vi "Configure Averaging.vi"(5 "Averaging State (F: Off)":bool, 7 "Channel (1)":i32=1, 8 "error in (no error)":errorcluster, 10 "Factor (16)":i32=16, 11 "VISA resource name":refnum<visa-resource-name>) -> (0 "error out":errorcluster, 3 "VISA resource name out":refnum<visa-resource-name>)   [LabVIEW 2011, in "Agilent ENA Series.lvlib"]
doc: "This VI configure the averaging for active channel."
uses:
  Agilent ENA Series.lvlib
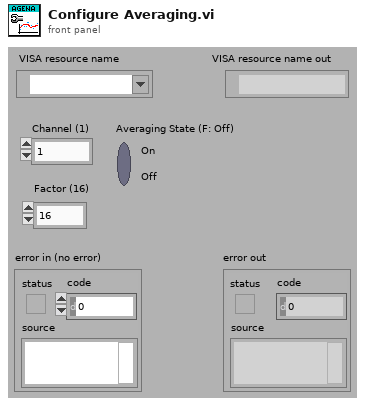
[diagram p1: front panel]
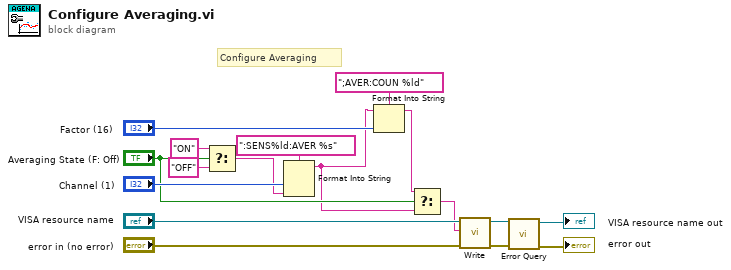
[diagram p0: block diagram]
diagram:
  # "Configure Averaging"
  n1 = Select(t="ON", s="Averaging State (F: Off)", f="OFF") -> (s? t:f=w11:string)
  n2 = Format Into String(format string=":SENS%ld:AVER %s", "Channel (1)", w11) -> (resulting string=w5:string)  [unwired: 2 in, 1 out]
  n3 = Format Into String(format string=";AVER:COUN %ld", initial string=w5, "Factor (16)") -> (resulting string=w7:string)  [unwired: 1 in, 1 out]
  n4 = Select(t=w7, s="Averaging State (F: Off)", f=w5) -> (s? t:f=w6:string)
  n5 = call "Write.vi"("error in (no error)"="error in (no error)", "String ()"=w6, "VISA resource name"="VISA resource name") -> ("error out"=w3:errorcluster, "VISA resource name out"=w4:refnum<visa-resource-name>)  [unwired: 6 in, 1 out]
  n6 = call "Error Query.vi"("error in (no error)"=w3, "VISA resource name"=w4) -> ("error out"=→"error out":errorcluster, "VISA resource name out"=→"VISA resource name out":refnum<visa-resource-name>)  [unwired: 6 in, 2 out]
